vi "GetCrateData.vi"(1 "Reverse?":bool, 3 "Type of scan":u16=1, 4 "save?":bool=TRUE, 5 "errorin":errorcluster, 6 "Array In":dbl[][](array[numeric]), 9 "Xmit Ring":i16, 10 "lines per plane":u16=128, 11 "Crate File Names":string[](array[string]), 12 "Syth Foc?":bool) -> (13 "Array":i16[][][](array[numeric]), 14 "Raw VGain (scale)":dbl, 15 "VGain (dB)":dbl[](array[numeric]), 18 "SA Data":dbl[][](array[numeric]), 19 "error out":errorcluster)   [LabVIEW 2022 SP3]
uses:
  Motion Controllers/-MotionRoutines/MotionGlobals.vi
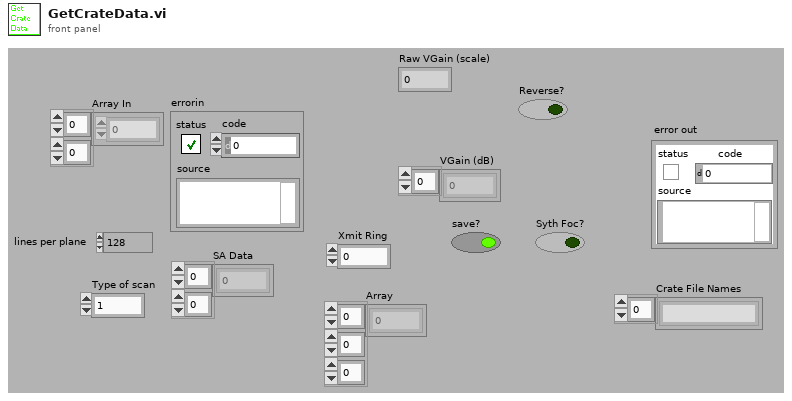
[diagram p1: front panel]
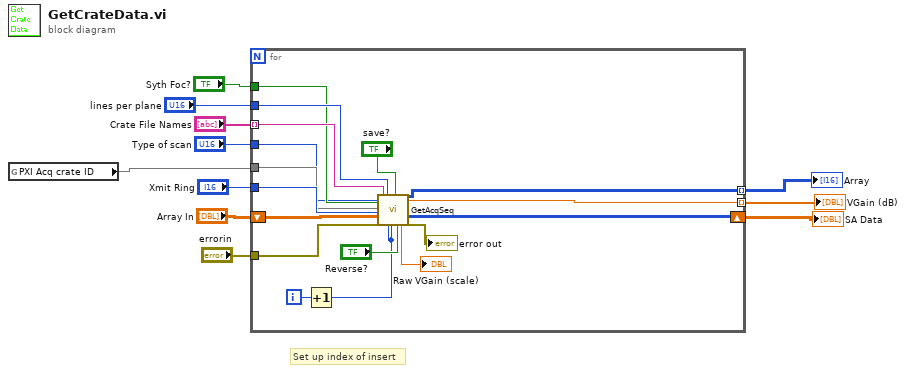
[diagram p0: block diagram]
diagram:
  # "Set up index of insert"
  n1 = global read "MotionGlobals.vi" "PXI Acq crate ID"() -> (w1)
  n2 = for {
    tunnel: [w17] -> w10 mode=indexing
    tunnel: "errorin" -> [w19]
    tunnel: "lines per plane" -> [w26]
    shift-right: [w15] -> w9
    shift-left: "Array In" -> [w21]
    tunnel: [w20] -> w7 mode=indexing
    tunnel: "Crate File Names" -> [w27] mode=indexing
    tunnel: "Syth Foc?" -> [w24]
    tunnel: "Xmit Ring" -> [w22]
    tunnel: w1 -> [w14]
    tunnel: "Type of scan" -> [w13]
    i -> [w28]
    n3 = Increment(x=w28) -> (x+1=w12:i32)
    n4 = call "GetAcqSeq.vi"("Digitizer Settings"=w13, "Acq Card ID"=w14, 4:w22, 5:w21, "errorin"=w19, "Numbered File"=w27, "lines per plane"=w26, "Channel (1)"=w12, "Rcv Ring"=w12, "save?"="save?", "Reverse?"="Reverse?", 16:w24) -> ("Raw VGain (scale)"=→"Raw VGain (scale)":dbl, "Array"=w20:i16[][], "VGain (dB)"=w17:dbl, "Synth App Out"=w15:i16[][], "error out"=→"error out":errorcluster)  [unwired: 4 in, 7 out]
  }
  "VGain (dB)" <- w10
  "SA Data" <- w9
  "Array" <- w7
